vi "Untitled 2.vi"() -> ()   [LabVIEW 2021]
uses:
  <instrlib>/Keithley 622x LV 2009/Utility/Typedefs/KE622x -- Instrument Type.ctl
  <instrlib>/Keithley 622x LV 2009/Configure/Source/Typedefs/KE622x -- Sweep Type.ctl
  <instrlib>/Keithley 622x LV 2009/Typedefs/KE622x -- On Off Control.ctl
  <instrlib>/Keithley 622x LV 2009/Configure/Trigger/Typedefs/KE622x -- Trig Layer Params.ctl
  <instrlib>/Keithley 622x LV 2009/Configure/Trigger/Low Level/Typedefs/KE622x -- Trig Source.ctl
  <instrlib>/Keithley 622x LV 2009/Configure/Trigger/Low Level/Typedefs/KE622x -- Trig Link Line.ctl
  <instrlib>/Keithley 622x LV 2009/Configure/Trigger/Low Level/Typedefs/KE622x -- Trig Output Mode.ctl
  <instrlib>/Keithley 622x LV 2009/Keithley 622x1.lvlib
panel:
  out "error out":errorcluster
  in  "error in (no error)":errorcluster
  in  "VISA resource name":refnum<visa-resource-name>
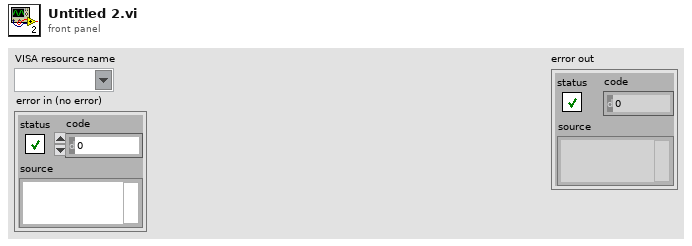
[diagram p1: front panel]
types:
  T1 = typedef "Keithley 622x1.lvlib/KE622x -- Trig Layer Params.ctl" = cluster{"Input Trig Source":T2, "Input Trig Link Line":T3, "Output Trig Mode":T4, "Output Trig Link Line":T3}
  T2 = typedef "Keithley 622x1.lvlib/KE622x -- Trig Source.ctl" = enum16{"Immediate", "Trigger Link"}
  T3 = typedef "Keithley 622x1.lvlib/KE622x -- Trig Link Line.ctl" = enum16{"1", "2", "3", "4", "5", "6"}
  T4 = typedef "Keithley 622x1.lvlib/KE622x -- Trig Output Mode.ctl" = enum16{"No Trig Out", "Source Turn On", "After Source Delay"}
  T5 = typedef "Keithley 622x1.lvlib/KE622x -- On Off Control.ctl" = enum16{"Off", "On"}
  T6 = typedef "Keithley 622x1.lvlib/KE622x -- Sweep Type.ctl" = enum16{"Linear", "Log", "List"}
  T7 = typedef "Keithley 622x1.lvlib/KE622x -- Instrument Type.ctl" = enum16{"KE6220", "KE6221"}
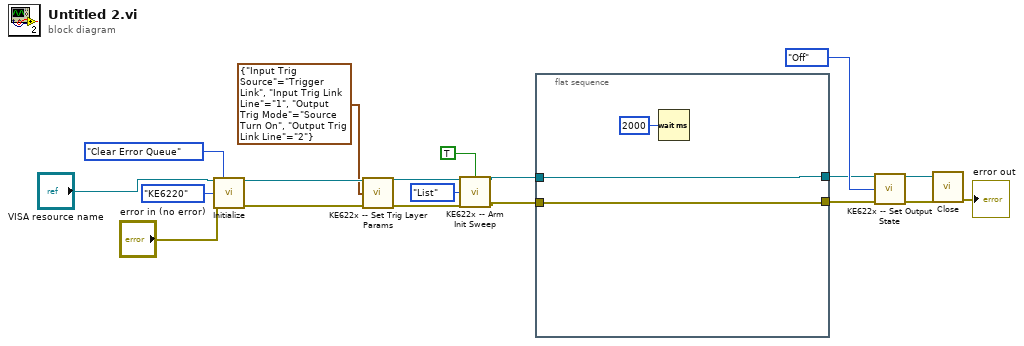
[diagram p0: block diagram]
diagram:
  n1 = call <instrlib>:"Initialize.vi"("VISA resource name"="VISA resource name", "Error Queue Option"=enum16{"Clear Error Queue", "Error Query"}."Clear Error Queue", "Instrument Type"=KE622x_--_Instrument_Type."KE6220", "error in (no error)"="error in (no error)") -> ("VISA resource name out"=w2:refnum<visa-resource-name>, "error out"=w3:errorcluster)  [unwired: 10 in]
  n2 = call <instrlib>:"KE622x -- Set Trig Layer Params.vi"("Resource In"=w2, "Trig Layer Params In"=T1 {"Input Trig Source"=enum."Trigger Link", "Input Trig Link Line"=enum."1", "Output Trig Mode"=enum."Source Turn On", "Output Trig Link Line"=enum."2"}, "error in (no error)"=w3) -> ("Resource Out (dupl)"=w5:refnum<visa-resource-name>, "error out"=w4:errorcluster)  [unwired: 10 in, 1 out]
  n3 = call <instrlib>:"KE622x -- Arm Init Sweep.vi"("Resource In"=w5, "Init Sweep? (T)"=TRUE, "Sweep Type"=KE622x_--_Sweep_Type."List", "error in (no error)"=w4) -> ("Resource Out (dupl)"=w7:refnum<visa-resource-name>, "error out"=w6:errorcluster)  [unwired: 10 in]
  n4 = flat-sequence {
    tunnel: w7 -> [w20]
    tunnel: [w21] -> w8
    tunnel: w6 -> [w21]
    tunnel: [w20] -> w9
    frame #0 {
      n5 = Wait (ms)(milliseconds to wait=u32 2000) -> ()  [unwired: 1 out]
    }
  }
  n6 = call <instrlib>:"KE622x -- Set Output State.vi"("Resource In"=w9, "Output State"=KE622x_--_On_Off_Control."Off", "error in (no error)"=w8) -> ("Resource Out (dupl)"=w11:refnum<visa-resource-name>, "error out"=w12:errorcluster)  [unwired: 11 in]
  n7 = call <instrlib>:"Close.vi"("VISA resource name"=w11, "error in (no error)"=w12) -> ("error out"=→"error out":errorcluster)  [unwired: 13 in]
